vi "PreOpenDevice.vi"(9 "Index":u32, 10 "type":u16(ring)=2 items=["USB-CAN"=2, "USB-CAN2.0"=3], 11 "param":T1[](array[typedef]) {"ACR0" format="%x"}) -> (1 "Channels":u32[](array[numeric]), 2 "DevIndex":u32, 3 "param out":T1[](array[typedef]) {"ACR0" format="%x"})   [LabVIEW 2011]
uses:
  Param.ctl
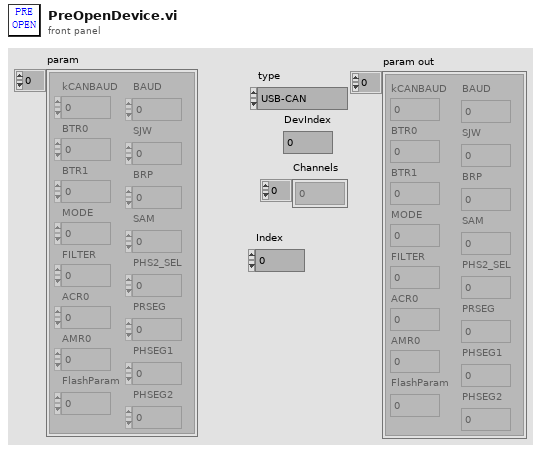
[diagram p1: front panel]
types:
  T1 = typedef "Param.ctl" = cluster{"kCANBAUD":u8, "BTR0":u8, "BTR1":u8, "MODE":u8, "FILTER":u8, "ACR0":u32, "AMR0":u32, "FlashParam":u32, "BAUD":u32, "SJW":u8, "BRP":u8, "SAM":u8, "PHS2_SEL":u8, "PRSEG":u8, "PHSEG1":u8, "PHSEG2":u8}
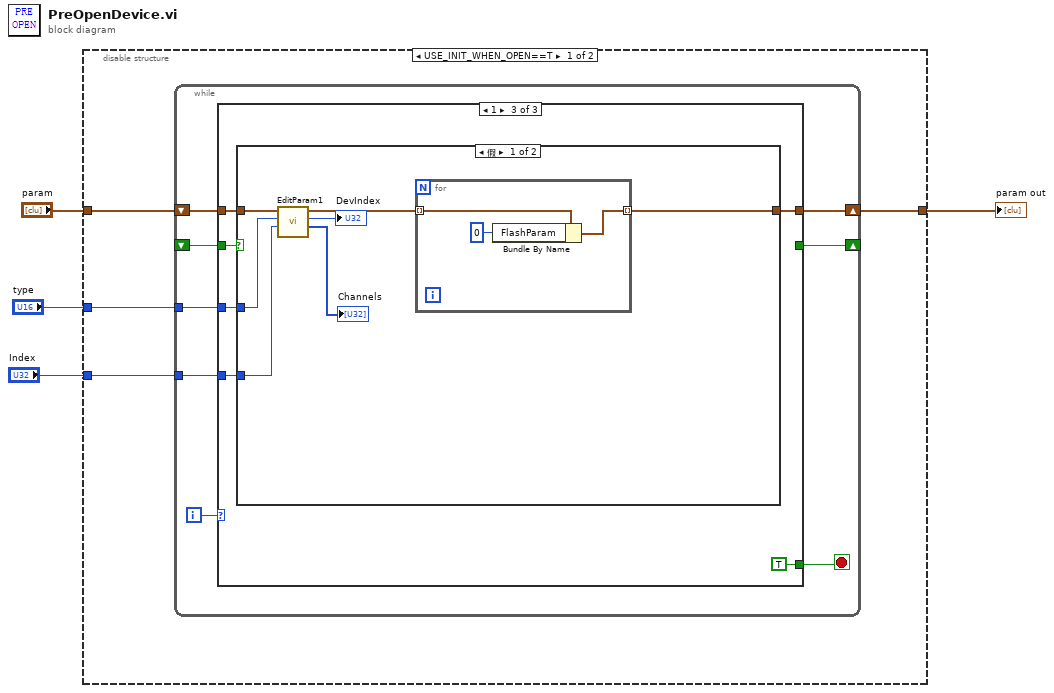
[diagram p0: block diagram]
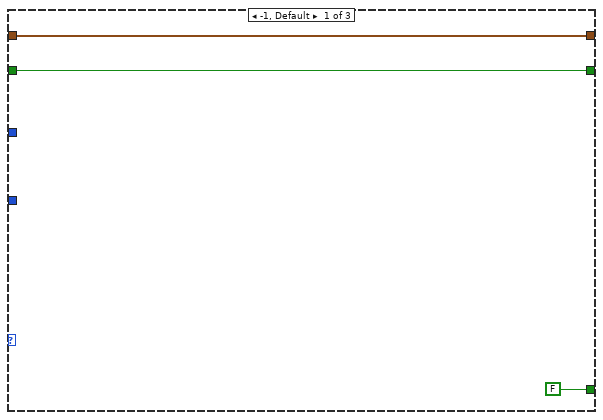
[diagram p2: hidden frame]
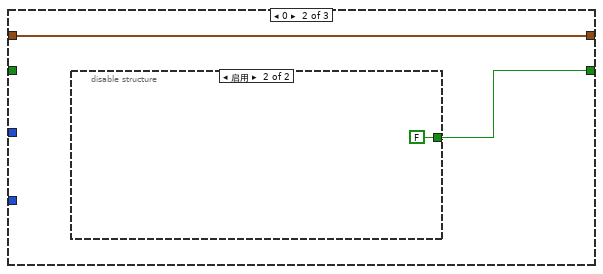
[diagram p3: hidden frame]
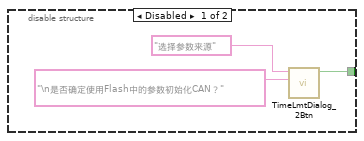
[diagram p4: hidden frame]
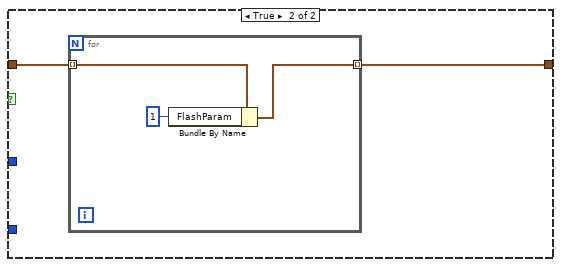
[diagram p5: hidden frame]
diagram:
  n1 = disable-structure shown="USE_INIT_WHEN_OPEN==T" {
    disable-tunnel: "param" -> [w8 w47]
    disable-tunnel: [w7 w47] -> w2
    disable-tunnel: "type" -> [w6 _]
    disable-tunnel: "Index" -> [w5 _]
    frame condition #0 (active) {
      n2 = while {
        shift-right: [w14] -> w7
        shift-left: w8 -> [w15]
        shift-right: [w12] -> _
        shift-left: _ -> [w11]
        tunnel: w6 -> [w10]
        tunnel: w5 -> [w9]
        i -> [w16]
        stop <- w13 stop-if-true
        n3 = case shown="1" w16 {
          tunnel: w15 -> [w19 w21 w30]
          tunnel: [w19 w21 w29] -> w14
          tunnel: [FALSE _ TRUE] -> w13
          tunnel: [w17 w20 _] -> w12
          tunnel: w11 -> [w17 _ w31]
          tunnel: w10 -> [_ _ w28]
          tunnel: w9 -> [_ _ w26]
          frame -1, Default {
          }
          frame 0 {
            n4 = disable-structure shown="启用" {
              disable-tunnel: [w22 FALSE ("OK?")] -> w20
              frame Disabled {
                n5 = call "TimeLmtDialog_2Btn.vi"("Infoin"="\n是否确定使用Flash中的参数初始化CAN？", "title"="选择参数来源") -> ("OK?"=w22:bool)  [unwired: 9 in]
              }
              frame Enabled {
              }
            }
          }
          frame 1 {
            n6 = case shown="假" w31 {
              tunnel: w30 -> [w38 w43]
              tunnel: [w36 w42] -> w29
              tunnel: w28 -> [w35 _]
              tunnel: w26 -> [w32 _]
              frame False {
                n7 = call "EditParam1.vi"("Index"=w32, "type"=w35, "param"=w38) -> ("Channels"=→"Channels":u32[], "DevIndex"=→"DevIndex":u32, "param out"=w37:T1[])  [unwired: 6 in]
                n8 = for {
                  tunnel: w37 -> [w41] mode=indexing
                  tunnel: [w40] -> w36 mode=indexing
                  n9 = Bundle By Name(cluster=w41, "FlashParam"=u32 0) -> (w40:T1)
                }
              }
              frame True {
                n10 = for {
                  tunnel: w43 -> [w46] mode=indexing
                  tunnel: [w44] -> w42 mode=indexing
                  n11 = Bundle By Name(cluster=w46, "FlashParam"=u32 1) -> (w44:T1)
                }
              }
            }
          }
        }
      }
    }
    frame condition #1 {
    }
  }
  "param out" <- w2
